vi "Aspect Ratio Score 2015.vi"(10 "Aspect Fudge Factor":dbl=1.0, 11 "Rectangle Array ltrb":dbl[](array[numeric])=[2.22, 1.4]) -> (2 "Short Edge Score":dbl, 3 "Long Edge Score":dbl)   [LabVIEW 2014]
doc: "Compare the ratio of the bounding box to that of the expected target. Score is in percent.\nFudge factor compensates for the cameras and camera modes that don't produce square pixels.\n\nSince inputs are particle measurements, the diagram doesn't expect to receive zero or negative values for either input."
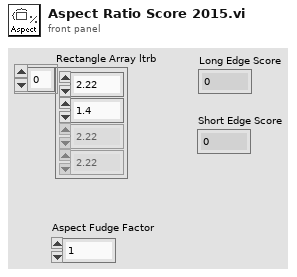
[diagram p1: front panel]
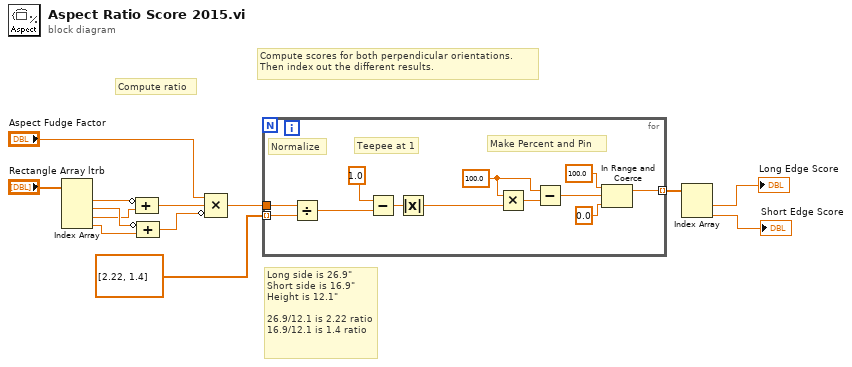
[diagram p0: block diagram]
diagram:
  # "Long side is 26.9\"\nShort side is 16.9\"\nHeight is 12.1\"\n\n26.9/12.1 is 2.22 ratio\n16.9/12.1 is 1.4 ratio"
  # "Compute scores for both perpendicular orientations.\nThen index out the different results."
  # "Compute ratio"
  n1 = Index Array(array="Rectangle Array ltrb") -> (element #1=w5:dbl, element #2=w8:dbl, element #3=w6:dbl, element #4=w7:dbl)  [unwired: 4 in]
  n2 = Compound Arithmetic op=ADD(invert w5, w6) -> (w4:dbl)
  n3 = Compound Arithmetic op=ADD(invert w8, w7) -> (w3:dbl)
  n4 = Compound Arithmetic op=MULTIPLY("Aspect Fudge Factor", w4, invert w3) -> (w13:dbl)
  n5 = for {
    tunnel: w13 -> [w15]
    tunnel: [w16] -> w11 mode=indexing
    tunnel: dbl[] [2.22, 1.4] -> [w14] mode=indexing
    w22 = 100.0 ("x/y")
    # "Make Percent and Pin"
    # "Teepee at 1"
    # "Normalize"
    n6 = Divide(x=w15, y=w14) -> (x/y=w24:dbl)
    n7 = Subtract(x=1.0 ("y"), y=w24) -> (x-y=w20:dbl)
    n8 = Absolute Value(x=w20) -> (abs(x)=w23:dbl)
    n9 = Multiply(x=w22, y=w23) -> (x*y=w25:dbl)
    n10 = Subtract(x=w22, y=w25) -> (x-y=w19:dbl)
    n11 = In Range and Coerce(upper limit=100.0, x=w19, lower limit=0.0) -> (coerced(x)=w16:dbl)  [unwired: 1 out]
  }
  n12 = Index Array(array=w11) -> (element #1=→"Long Edge Score":dbl, element #2=→"Short Edge Score":dbl)  [unwired: 2 in]
